vi "InstallPlugins.vi"() -> ()   [LabVIEW 2014]
panel:
  out "error out":errorcluster
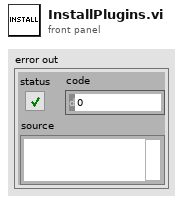
[diagram p1: front panel]
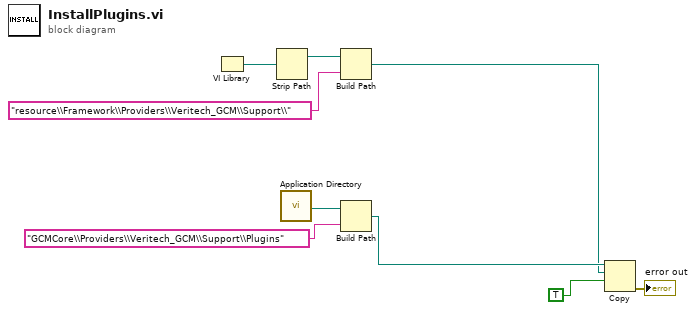
[diagram p0: block diagram]
diagram:
  n1 = VI Library() -> (path=w7:path)
  n2 = Strip Path(path=w7) -> (stripped path=w6:path)  [unwired: 1 out]
  n3 = call <vilib>:"Application Directory.vi"() -> ("Application Directory"=w9:path)
  n4 = Build Path(base path=w6, name or relative path="resource\\Framework\\Providers\\Veritech_GCM\\Support\\") -> (appended path=w1:path)
  n5 = Build Path(base path=w9, name or relative path="GCMCore\\Providers\\Veritech_GCM\\Support\\Plugins") -> (appended path=w2:path)
  n6 = Copy(9:TRUE ("overwrite (F)"), 10:w1, 11:w2) -> (0:→"error out":errorcluster)  [unwired: 2 in, 2 out]
